vi "DEMO.vi"() -> ()   [LabVIEW 2011, in "BMP File.lvlib"]
uses:
  BMP File.lvlib
panel:
  out "new picture":picture caption="新图片"
  in  "文件（使用对话框）":path
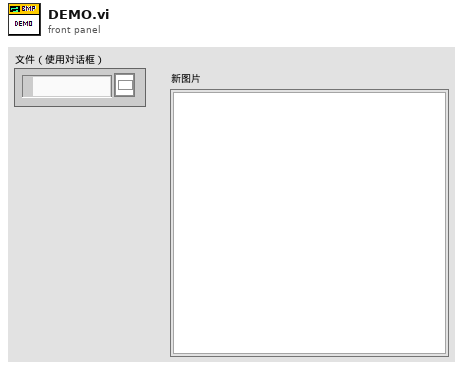
[diagram p1: front panel]
types:
  T1 = typedef "imagedata.ctl" = cluster{"image type":i32, "image depth":i32, "image":u8[], "mask":u8[], "colors":u32[], "Rectangle":cluster{"left":i16, "top":i16, "right":i16, "bottom":i16}}
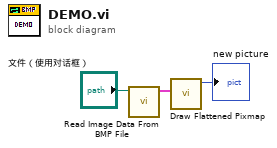
[diagram p0: block diagram]
diagram:
  n1 = call "Read Image Data From BMP File.vi"("文件（使用对话框）"="文件（使用对话框）") -> ("Image Data"=w2:T1)  [unwired: 9 in, 1 out]
  n2 = call <vilib>:"Draw Flattened Pixmap.vi"("image data"=w2) -> ("new picture"=→"new picture":picture)  [unwired: 8 in]
